vi "GetAprilTags.vi"(7 "Using 3D Targeting":bool=TRUE) -> (0 "Lemon AprilTag Data [t-?]":dbl[](array[numeric]), 1 "Lemon Vision Target Valid [t-?]":bool, 2 "Lime AprilTag Data [t-?]":dbl[](array[numeric]), 3 "Lime Vision Target Valid [t-?]":bool, 4 "Lemon Vision Timestamp (ms)":u32, 6 "Lime Vision Timestamp (ms)":u32)   [LabVIEW 2023]
doc: "Reads the raw data from the LimeLight camera assigned to detecting AprilTags. Performs some minor transformations, conducts intial validity checks, and estimates the vision data timestamp."
uses:
  2d64956e-cf35-4d84-838e-e30eff74bf58.vi
  90f2414f-78bc-452b-a638-30c28710607a.vi
  <vilib>/Rock Robotics/Network Tables/NT Read Number.vi
  GlobalDriverStationData.vi
  <vilib>/Rock Robotics/Network Tables/NT Read Numeric Array.vi
  GlobalPoseAndTargeting.vi
  8fc9d911-d6d4-4d98-b6c3-957ea94c93cf.vi
  832ec9d1-ff64-4476-b10f-783a12dcd09d.vi
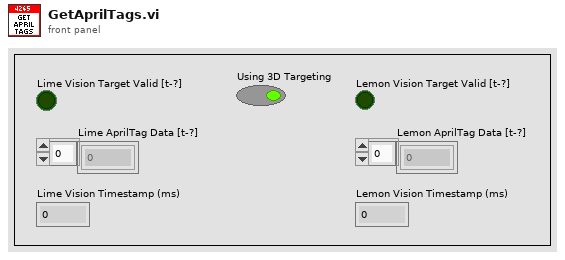
[diagram p1: front panel]
types:
  T1 = enum16{"Boot Up", "Camera Override", "HUB Targeting", "CARGO Tracking"}
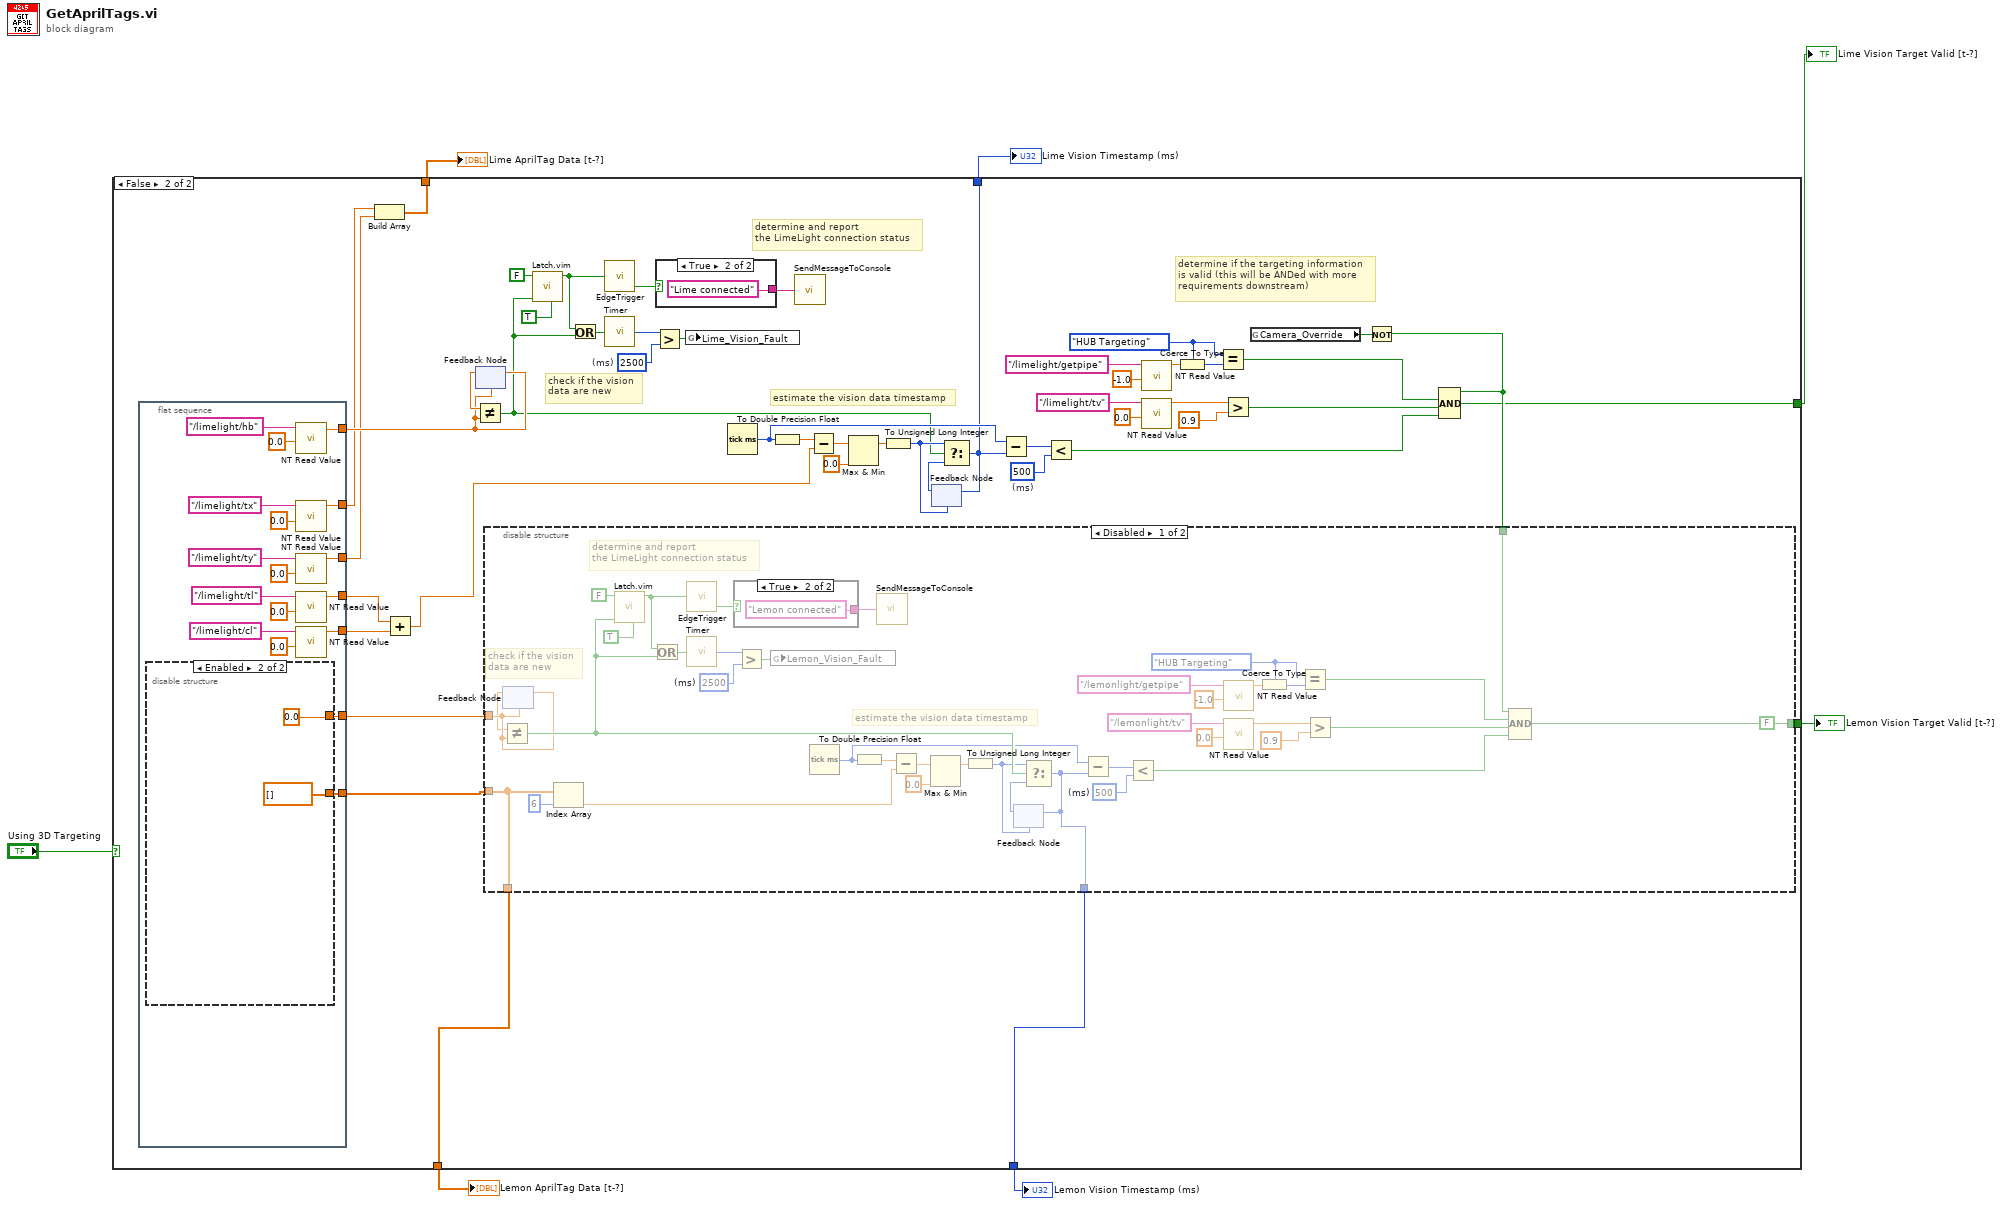
[diagram p0: block diagram]
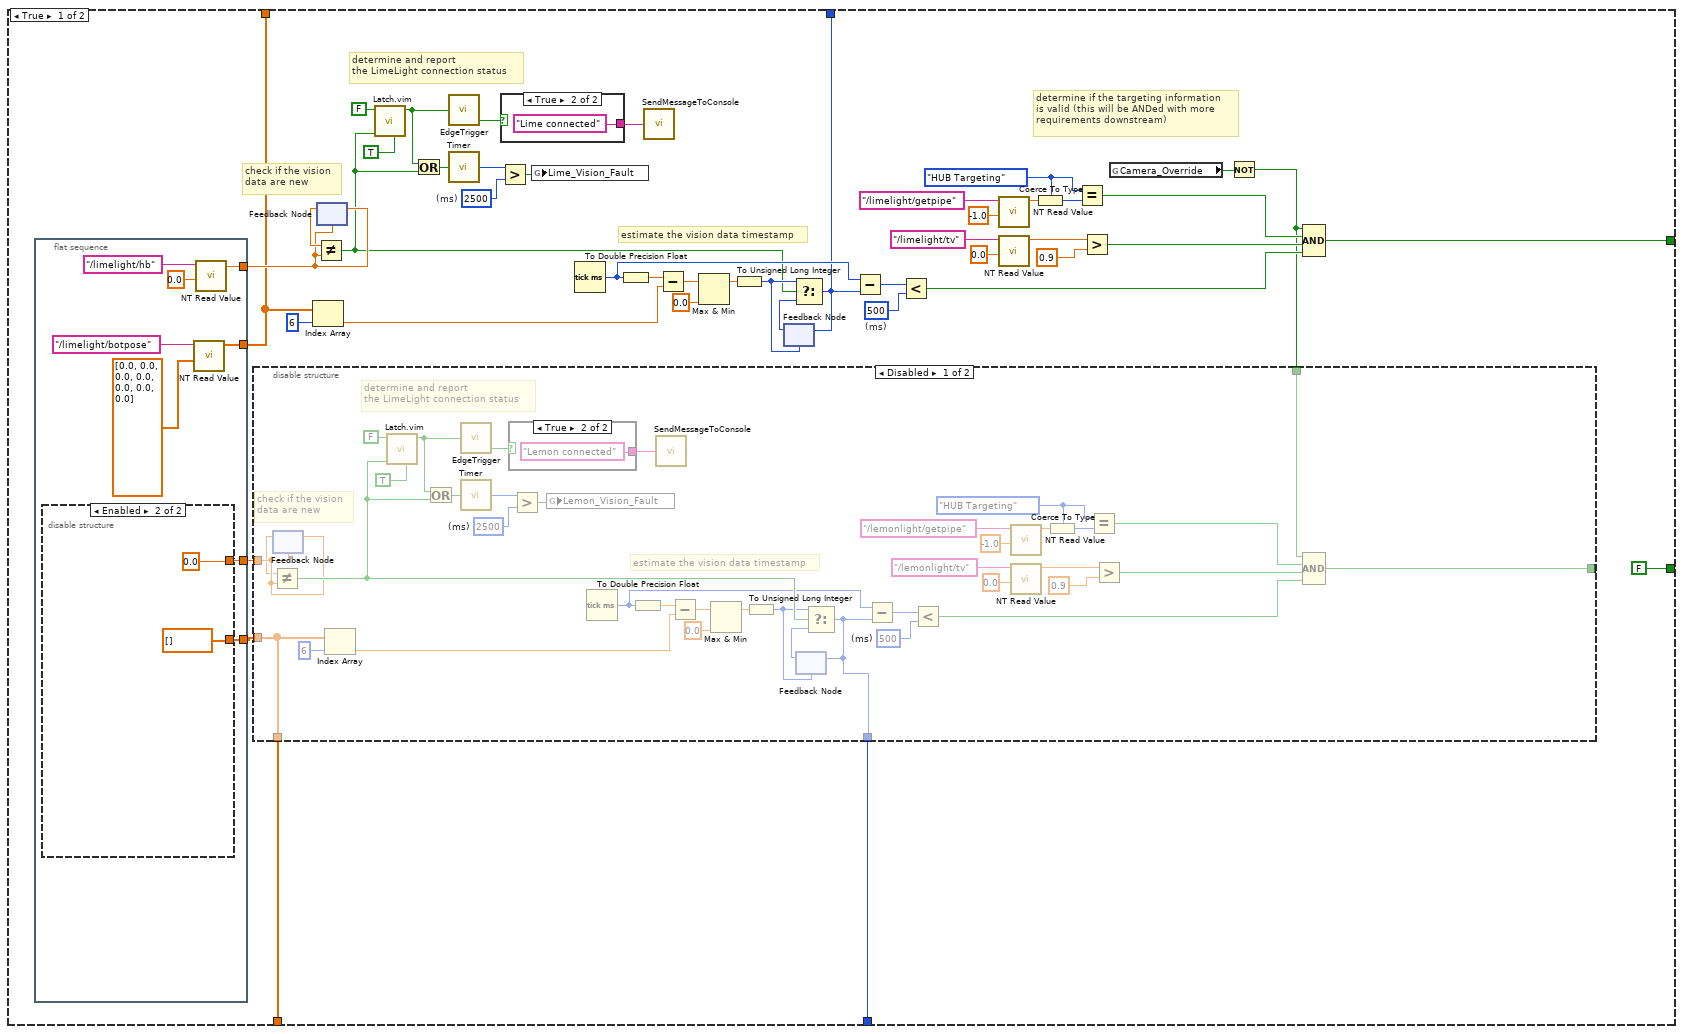
[diagram p2: hidden frame]
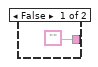
[diagram p3: hidden frame]
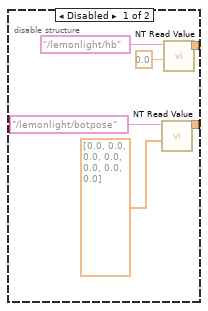
[diagram p5: hidden frame]
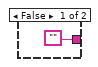
[diagram p6: hidden frame]
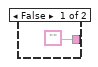
[diagram p7: hidden frame]
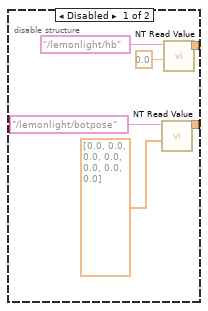
[diagram p9: hidden frame]
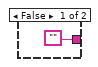
[diagram p10: hidden frame]
diagram:
  n1 = case shown="False" "Using 3D Targeting" {
    tunnel: [w13 w122] -> w7
    tunnel: [w12 w121] -> w6
    tunnel: [w11 w115] -> w5
    tunnel: [FALSE FALSE] -> w3
    tunnel: [w9 w119] -> w2
    tunnel: [w8 w118] -> w1
    frame True {
      w29 = u32 2500  # (ms)
      w22 = u32 500  # (ms)
      w43 = T1."HUB Targeting" ("x")
      # "determine and report\nthe LimeLight connection status"
      # "determine if the targeting information\nis valid (this will be ANDed with more\nrequirements downstream)"
      # "estimate the vision data timestamp"
      # "check if the vision\ndata are new"
      n2 = flat-sequence {
        tunnel: [w99] -> w20
        tunnel: [w96] -> w11
        tunnel: [w95] -> w16
        tunnel: [w94] -> w15
        frame #0 {
          n3 = disable-structure shown="Enabled" {
            disable-tunnel: [w103 dbl[] [] ("value")] -> w95
            disable-tunnel: [w102 0.0 ("value")] -> w94
            frame Disabled {
              n4 = call-poly <vilib>:"NT Read Value.vi"("default value"=dbl[] [0.0, 0.0, 0.0, 0.0, 0.0, 0.0, 0.0], "name"="/lemonlight/botpose" ("Name")) -> ("value"=w103:dbl[])  [unwired: 7 in, 2 out]
              n5 = call-poly <vilib>:"NT Read Value.vi"("default value"=0.0 ("Default Value"), "name"="/lemonlight/hb" ("Name")) -> ("value"=w102:dbl)  [unwired: 7 in, 2 out]
            }
            frame Enabled {
            }
          }
          n6 = call-poly <vilib>:"NT Read Value.vi"("default value"=dbl[] [0.0, 0.0, 0.0, 0.0, 0.0, 0.0, 0.0], "name"="/limelight/botpose" ("Name")) -> ("value"=w96:dbl[])  [unwired: 7 in, 2 out]
          n7 = call-poly <vilib>:"NT Read Value.vi"("default value"=0.0 ("Default Value"), "name"="/limelight/hb" ("Name")) -> ("value"=w99:dbl)  [unwired: 7 in, 2 out]
        }
      }
      n8 = Index Array(array=w11, index=6) -> (element=w17:dbl)
      n9 = feedback #1(w20) -> (w31:dbl)
      n10 = Not Equal?(x=w31, y=w20) -> (x != y?=w19:bool)
      n11 = feedback-in #1(w20) -> ()
      n12 = call "Latch.vim"("Default Value"=TRUE, "Latch Signal"=w19, "Latch Value"=FALSE) -> ("Latched"=w25:bool)  [unwired: 8 in]
      n13 = Or(x=w25, y=w19) -> (x .or. y?=w28:bool)
      n14 = call "EdgeTrigger.vi"("Input Signal"=w25) -> ("Falling Edge Trigger"=w23:bool)  [unwired: 2 out]
      n15 = call "Timer.vi"("Reset Timer"=w28) -> ("Time (ms)"=w30:u32)
      n16 = Greater?(x=w30, y=w29) -> (0:w21:bool)
      n17 = case shown="True" w23 {
        tunnel: ["" "Lime connected" ("Message")] -> w24
        frame False {
        }
        frame True {
        }
      }
      n18 = global write "GlobalPoseAndTargeting.vi" "Lime_Vision_Fault"(w21) -> ()
      n19 = Tick Count (ms)() -> (millisecond timer value=w35:u32)
      n20 = To Double Precision Float(number=w35) -> (double precision float=w40:dbl)
      n21 = call "SendMessageToConsole.vi"("Message String"=w24) -> ()  [unwired: 1 in]
      n22 = Subtract(x=w40, y=w17) -> (x-y=w39:dbl)
      n23 = Max & Min(x=w39, y=0.0) -> (max(x,y)=w37:dbl)  [unwired: 1 out]
      n24 = To Unsigned Long Integer(number=w37) -> (unsigned 32bit integer=w36:u32)
      n25 = feedback #2(w36) -> (w41:u32)
      n26 = Select(t=w36, s=w19, f=w41) -> (s? t:f=w12:u32)
      n27 = feedback-in #2(w12) -> ()
      n28 = Subtract(x=w35, y=w12) -> (x-y=w34:u32)
      n29 = Less?(x=w34, y=w22) -> (x < y?=w33:bool)
      n30 = call-poly <vilib>:"NT Read Value.vi"("default value"=-1.0 ("Default Value"), "name"="/limelight/getpipe" ("Name")) -> ("value"=w46:dbl)  [unwired: 7 in, 2 out]
      n31 = call-poly <vilib>:"NT Read Value.vi"("default value"=0.0 ("Default Value"), "name"="/limelight/tv" ("Name")) -> ("value"=w52:dbl)  [unwired: 7 in, 2 out]
      n32 = Coerce To Type(0:w46, 1:w43) -> (2:w45:T1)
      n33 = Equal?(x=w43, y=w45) -> (x = y?=w44:bool)
      n34 = Greater?(x=w52, y=0.9) -> (0:w42:bool)
      n35 = global read "GlobalDriverStationData.vi" "Camera_Override"() -> (w32:bool)
      n36 = Not(x=w32) -> (.not. x?=w14:bool)
      n37 = disable-structure shown="Disabled" {
        disable-tunnel: w16 -> [w53 _]
        disable-tunnel: w15 -> [w58 _]
        disable-tunnel: w14 -> [w56 _]
        disable-tunnel: [w55 _] -> _
        disable-tunnel: [w54 _] -> w9
        disable-tunnel: [w53 _] -> w8
        frame Disabled {
          w80 = u32 2500  # (ms)
          w87 = u32 500  # (ms)
          w68 = T1."HUB Targeting" ("x")
          # "determine and report\nthe LimeLight connection status"
          # "estimate the vision data timestamp"
          # "check if the vision\ndata are new"
          n38 = feedback #3(w58) -> (w57:dbl)
          n39 = Not Equal?(x=w57, y=w58) -> (x != y?=w89:bool)
          n40 = feedback-in #3(w58) -> ()
          n41 = Index Array(array=w53, index=6) -> (element=w91:dbl)
          n42 = call "Latch.vim"("Default Value"=TRUE, "Latch Signal"=w89, "Latch Value"=FALSE) -> ("Latched"=w84:bool)  [unwired: 8 in]
          n43 = Or(x=w84, y=w89) -> (x .or. y?=w81:bool)
          n44 = call "EdgeTrigger.vi"("Input Signal"=w84) -> ("Falling Edge Trigger"=w86:bool)  [unwired: 2 out]
          n45 = call "Timer.vi"("Reset Timer"=w81) -> ("Time (ms)"=w79:u32)
          n46 = case shown="True" w86 {
            tunnel: ["" "Lemon connected" ("Message")] -> w85
            frame False {
            }
            frame True {
            }
          }
          n47 = Greater?(x=w79, y=w80) -> (0:w88:bool)
          n48 = global write "GlobalPoseAndTargeting.vi" "Lemon_Vision_Fault"(w88) -> ()
          n49 = Tick Count (ms)() -> (millisecond timer value=w76:u32)
          n50 = To Double Precision Float(number=w76) -> (double precision float=w71:dbl)
          n51 = call "SendMessageToConsole.vi"("Message String"=w85) -> ()  [unwired: 1 in]
          n52 = Subtract(x=w71, y=w91) -> (x-y=w72:dbl)
          n53 = Max & Min(x=w72, y=0.0) -> (max(x,y)=w74:dbl)  [unwired: 1 out]
          n54 = To Unsigned Long Integer(number=w74) -> (unsigned 32bit integer=w75:u32)
          n55 = feedback #4(w75) -> (w70:u32)
          n56 = Select(t=w75, s=w89, f=w70) -> (s? t:f=w54:u32)
          n57 = feedback-in #4(w54) -> ()
          n58 = Subtract(x=w76, y=w54) -> (x-y=w77:u32)
          n59 = Less?(x=w77, y=w87) -> (x < y?=w78:bool)
          n60 = call-poly <vilib>:"NT Read Value.vi"("default value"=-1.0 ("Default Value"), "name"="/lemonlight/getpipe" ("Name")) -> ("value"=w65:dbl)  [unwired: 7 in, 2 out]
          n61 = call-poly <vilib>:"NT Read Value.vi"("default value"=0.0 ("Default Value"), "name"="/lemonlight/tv" ("Name")) -> ("value"=w59:dbl)  [unwired: 7 in, 2 out]
          n62 = Coerce To Type(0:w65, 1:w68) -> (2:w66:T1)
          n63 = Equal?(x=w68, y=w66) -> (x = y?=w67:bool)
          n64 = Greater?(x=w59, y=0.9) -> (0:w69:bool)
          n65 = Compound Arithmetic op=AND(w56, w67, w69, w78) -> (w55:bool)
        }
        frame Enabled {
        }
      }
      n66 = Compound Arithmetic op=AND(w14, w44, w42, w33) -> (w13:bool)
    }
    frame False {
      w136 = u32 2500  # (ms)
      w129 = u32 500  # (ms)
      w150 = T1."HUB Targeting" ("x")
      # "determine and report\nthe LimeLight connection status"
      # "determine if the targeting information\nis valid (this will be ANDed with more\nrequirements downstream)"
      # "estimate the vision data timestamp"
      # "check if the vision\ndata are new"
      n67 = flat-sequence {
        tunnel: [w215] -> w127
        tunnel: [w212] -> w117
        tunnel: [w214] -> w125
        tunnel: [w213] -> w124
        tunnel: [w208] -> w113
        tunnel: [w207] -> w116
        tunnel: [w205] -> w114
        frame #0 {
          n68 = disable-structure shown="Enabled" {
            disable-tunnel: [w219 dbl[] [] ("value")] -> w214
            disable-tunnel: [w218 0.0 ("value")] -> w213
            frame Disabled {
              n69 = call-poly <vilib>:"NT Read Value.vi"("default value"=dbl[] [0.0, 0.0, 0.0, 0.0, 0.0, 0.0, 0.0], "name"="/lemonlight/botpose" ("Name")) -> ("value"=w219:dbl[])  [unwired: 7 in, 2 out]
              n70 = call-poly <vilib>:"NT Read Value.vi"("default value"=0.0 ("Default Value"), "name"="/lemonlight/hb" ("Name")) -> ("value"=w218:dbl)  [unwired: 7 in, 2 out]
            }
            frame Enabled {
            }
          }
          n71 = call-poly <vilib>:"NT Read Value.vi"("default value"=0.0 ("Default Value"), "name"="/limelight/hb" ("Name")) -> ("value"=w215:dbl)  [unwired: 7 in, 2 out]
          n72 = call-poly <vilib>:"NT Read Value.vi"("default value"=0.0, "name"="/limelight/tx" ("Name")) -> ("value"=w212:dbl)  [unwired: 7 in, 2 out]
          n73 = call-poly <vilib>:"NT Read Value.vi"("default value"=0.0, "name"="/limelight/ty" ("Name")) -> ("value"=w207:dbl)  [unwired: 7 in, 2 out]
          n74 = call-poly <vilib>:"NT Read Value.vi"("default value"=0.0, "name"="/limelight/tl" ("Name")) -> ("value"=w208:dbl)  [unwired: 7 in, 2 out]
          n75 = call-poly <vilib>:"NT Read Value.vi"("default value"=0.0, "name"="/limelight/cl" ("Name")) -> ("value"=w205:dbl)  [unwired: 7 in, 2 out]
        }
      }
      n76 = Build Array(w117, w116) -> (w115:dbl[])
      n77 = Add(x=w113, y=w114) -> (x+y=w112:dbl)
      n78 = feedback #5(w127) -> (w138:dbl)
      n79 = Not Equal?(x=w138, y=w127) -> (x != y?=w126:bool)
      n80 = feedback-in #5(w127) -> ()
      n81 = call "Latch.vim"("Default Value"=TRUE, "Latch Signal"=w126, "Latch Value"=FALSE) -> ("Latched"=w132:bool)  [unwired: 8 in]
      n82 = Or(x=w132, y=w126) -> (x .or. y?=w135:bool)
      n83 = call "EdgeTrigger.vi"("Input Signal"=w132) -> ("Falling Edge Trigger"=w130:bool)  [unwired: 2 out]
      n84 = call "Timer.vi"("Reset Timer"=w135) -> ("Time (ms)"=w137:u32)
      n85 = Greater?(x=w137, y=w136) -> (0:w128:bool)
      n86 = case shown="True" w130 {
        tunnel: ["" "Lime connected" ("Message")] -> w131
        frame False {
        }
        frame True {
        }
      }
      n87 = global write "GlobalPoseAndTargeting.vi" "Lime_Vision_Fault"(w128) -> ()
      n88 = Tick Count (ms)() -> (millisecond timer value=w142:u32)
      n89 = To Double Precision Float(number=w142) -> (double precision float=w147:dbl)
      n90 = call "SendMessageToConsole.vi"("Message String"=w131) -> ()  [unwired: 1 in]
      n91 = Subtract(x=w147, y=w112) -> (x-y=w146:dbl)
      n92 = Max & Min(x=w146, y=0.0) -> (max(x,y)=w144:dbl)  [unwired: 1 out]
      n93 = To Unsigned Long Integer(number=w144) -> (unsigned 32bit integer=w143:u32)
      n94 = feedback #6(w143) -> (w148:u32)
      n95 = Select(t=w143, s=w126, f=w148) -> (s? t:f=w121:u32)
      n96 = feedback-in #6(w121) -> ()
      n97 = Subtract(x=w142, y=w121) -> (x-y=w141:u32)
      n98 = Less?(x=w141, y=w129) -> (x < y?=w140:bool)
      n99 = call-poly <vilib>:"NT Read Value.vi"("default value"=-1.0 ("Default Value"), "name"="/limelight/getpipe" ("Name")) -> ("value"=w153:dbl)  [unwired: 7 in, 2 out]
      n100 = call-poly <vilib>:"NT Read Value.vi"("default value"=0.0 ("Default Value"), "name"="/limelight/tv" ("Name")) -> ("value"=w159:dbl)  [unwired: 7 in, 2 out]
      n101 = Coerce To Type(0:w153, 1:w150) -> (2:w152:T1)
      n102 = Equal?(x=w150, y=w152) -> (x = y?=w151:bool)
      n103 = Greater?(x=w159, y=0.9) -> (0:w149:bool)
      n104 = global read "GlobalDriverStationData.vi" "Camera_Override"() -> (w139:bool)
      n105 = Not(x=w139) -> (.not. x?=w123:bool)
      n106 = disable-structure shown="Disabled" {
        disable-tunnel: w125 -> [w160 _]
        disable-tunnel: w124 -> [w165 _]
        disable-tunnel: w123 -> [w163 _]
        disable-tunnel: [w162 _] -> _
        disable-tunnel: [w161 _] -> w119
        disable-tunnel: [w160 _] -> w118
        frame Disabled {
          w187 = u32 2500  # (ms)
          w194 = u32 500  # (ms)
          w175 = T1."HUB Targeting" ("x")
          # "determine and report\nthe LimeLight connection status"
          # "estimate the vision data timestamp"
          # "check if the vision\ndata are new"
          n107 = feedback #7(w165) -> (w164:dbl)
          n108 = Not Equal?(x=w164, y=w165) -> (x != y?=w196:bool)
          n109 = feedback-in #7(w165) -> ()
          n110 = Index Array(array=w160, index=6) -> (element=w198:dbl)
          n111 = call "Latch.vim"("Default Value"=TRUE, "Latch Signal"=w196, "Latch Value"=FALSE) -> ("Latched"=w191:bool)  [unwired: 8 in]
          n112 = Or(x=w191, y=w196) -> (x .or. y?=w188:bool)
          n113 = call "EdgeTrigger.vi"("Input Signal"=w191) -> ("Falling Edge Trigger"=w193:bool)  [unwired: 2 out]
          n114 = call "Timer.vi"("Reset Timer"=w188) -> ("Time (ms)"=w186:u32)
          n115 = case shown="True" w193 {
            tunnel: ["" "Lemon connected" ("Message")] -> w192
            frame False {
            }
            frame True {
            }
          }
          n116 = Greater?(x=w186, y=w187) -> (0:w195:bool)
          n117 = global write "GlobalPoseAndTargeting.vi" "Lemon_Vision_Fault"(w195) -> ()
          n118 = Tick Count (ms)() -> (millisecond timer value=w183:u32)
          n119 = To Double Precision Float(number=w183) -> (double precision float=w178:dbl)
          n120 = call "SendMessageToConsole.vi"("Message String"=w192) -> ()  [unwired: 1 in]
          n121 = Subtract(x=w178, y=w198) -> (x-y=w179:dbl)
          n122 = Max & Min(x=w179, y=0.0) -> (max(x,y)=w181:dbl)  [unwired: 1 out]
          n123 = To Unsigned Long Integer(number=w181) -> (unsigned 32bit integer=w182:u32)
          n124 = feedback #8(w182) -> (w177:u32)
          n125 = Select(t=w182, s=w196, f=w177) -> (s? t:f=w161:u32)
          n126 = feedback-in #8(w161) -> ()
          n127 = Subtract(x=w183, y=w161) -> (x-y=w184:u32)
          n128 = Less?(x=w184, y=w194) -> (x < y?=w185:bool)
          n129 = call-poly <vilib>:"NT Read Value.vi"("default value"=-1.0 ("Default Value"), "name"="/lemonlight/getpipe" ("Name")) -> ("value"=w172:dbl)  [unwired: 7 in, 2 out]
          n130 = call-poly <vilib>:"NT Read Value.vi"("default value"=0.0 ("Default Value"), "name"="/lemonlight/tv" ("Name")) -> ("value"=w166:dbl)  [unwired: 7 in, 2 out]
          n131 = Coerce To Type(0:w172, 1:w175) -> (2:w173:T1)
          n132 = Equal?(x=w175, y=w173) -> (x = y?=w174:bool)
          n133 = Greater?(x=w166, y=0.9) -> (0:w176:bool)
          n134 = Compound Arithmetic op=AND(w163, w174, w176, w185) -> (w162:bool)
        }
        frame Enabled {
        }
      }
      n135 = Compound Arithmetic op=AND(w123, w151, w149, w140) -> (w122:bool)
    }
  }
  "Lime Vision Target Valid [t-?]" <- w7
  "Lime Vision Timestamp (ms)" <- w6
  "Lime AprilTag Data [t-?]" <- w5
  "Lemon Vision Target Valid [t-?]" <- w3
  "Lemon Vision Timestamp (ms)" <- w2
  "Lemon AprilTag Data [t-?]" <- w1
